vi "GV FIFO OUT gate.vi"() -> ()   [LabVIEW 2017]
panel:
  out "FIFO OUT gate":bool
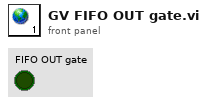
[diagram p1: front panel]
diagram:
